vi "Replace HDI Precheck.vi"(8 "error in":errorcluster, 9 "Slot Number in":i32, 10 "Chuck Number in":i32, 11 "PickupTool Class in":refnum<class "PickerTool Class.lvclass">) -> (0 "error out":errorcluster, 3 "PickupTool Class out":refnum<class "PickerTool Class.lvclass">)   [LabVIEW 2011, in "PickerTool Class.lvclass"]
uses:
  PickerTool Class.lvclass
  PickerTool Class.lvclass/PickerTool Class.ctl
  WorkTable Class/WorkTable Class.lvclass
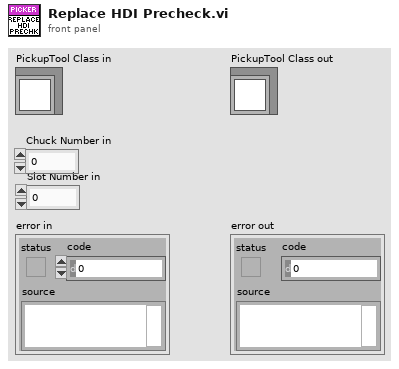
[diagram p1: front panel]
types:
  T1 = enum16{"Empty", "Unglued", "Stamped", "PartOnTop", "Weighted", "Unpotted", "Potted"}
  T2 = typedef "Worktable_Module Slot.ctl" = cluster{"Slot State":enum16{"Empty", "Unglued", "Stamped", "PartOnTop", "Weighted", "Unpotted", "Potted"}, "BBM Type":enum16{"None", "BBM", "GlassSlide"}, "HDI Type":enum16{"None", "HDI", "Polyimide"}, "Vacuum Channel":u8, "Location/Orientation BBM":T3, "Location/Orientation HDI":T3, "S/N":string}
  T3 = typedef "Position_Orientation.ctl" = cluster{"Center":refnum<class "Vec3d Class.lvclass">, "Orientation":refnum<class "Orient3d Class.lvclass">}
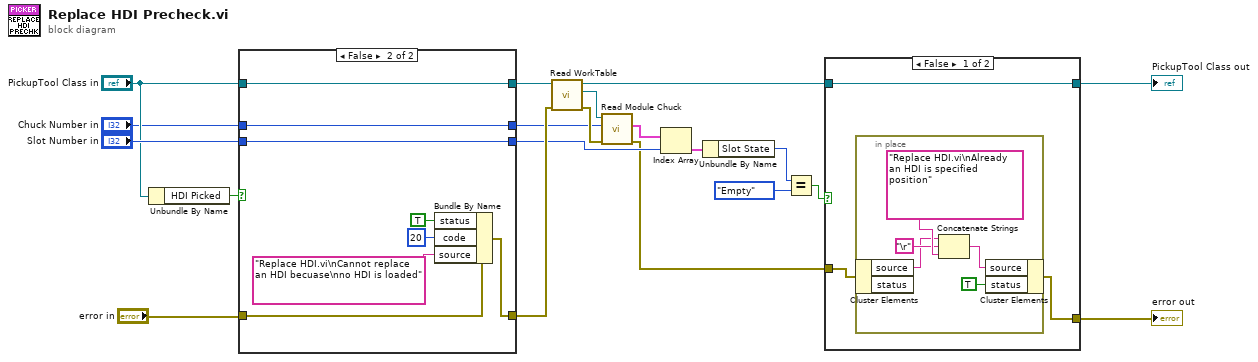
[diagram p0: block diagram]
diagram:
  n1 = Unbundle By Name("PickupTool Class in") -> ("HDI Picked"=w13:bool)
  n2 = case shown="False" w13 {
    tunnel: "PickupTool Class in" -> [w24 w32]
    tunnel: "error in" -> [w23 w31]
    tunnel: [w24 w32] -> w15
    tunnel: [w23 w27] -> w16
    tunnel: "Slot Number in" -> [w22 w26]
    tunnel: [w22 w26] -> w6
    tunnel: "Chuck Number in" -> [w21 w25]
    tunnel: [w21 w25] -> w8
    frame True {
    }
    frame False {
      n3 = Bundle By Name(cluster=w31, "status"=TRUE, "code"=20, "source"="Replace HDI.vi\nCannot replace an HDI becuase\nno HDI is loaded") -> (w27:errorcluster)
    }
  }
  n4 = call-dynamic "Read WorkTable.vi"("error in"=w16, "Gantry Class in"=w15) -> ("error out"=w10:errorcluster, "WorkTable Class.lvclass"=w9:refnum<class "WorkTable Class.lvclass">, "Gantry Class out"=w19:refnum<class "PickerTool Class.lvclass">)  [unwired: 7 in]
  n5 = call-dynamic "Read Module Chuck.vi"("error in"=w10, "index"=w8, "WorkTable in"=w9) -> ("error out"=w2:errorcluster, "Module Slots"=w7:T2[])  [unwired: 6 in, 1 out]
  n6 = Index Array(array=w7, index=w6) -> (element=w5:T2)
  n7 = Unbundle By Name(w5) -> ("Slot State"=w4:T1)
  n8 = Equal?(x=w4, y=T1."Empty" ("Slot State")) -> (x = y?=w18:bool)
  n9 = case shown="False" w18 {
    tunnel: w19 -> [w34 w42]
    tunnel: [w35 w41] -> w1
    tunnel: [w34 w42] -> w20
    tunnel: w2 -> [w33 w41]
    frame False {
      n10 = in-place {
        n11 = in-place-cluster #1(w33) -> ("source"=w37:string)  [unwired: 1 out]
        n12 = Concatenate Strings(w37, "\r", "Replace HDI.vi\nAlready an HDI is specified position" ("string")) -> (w38:string)
        n13 = in-place-cluster #1("source"=w38, "status"=TRUE) -> (w35:errorcluster)
      }
    }
    frame True {
    }
  }
  "error out" <- w1
  "PickupTool Class out" <- w20
